vi "Parametros de adquisición texto para main.vi"(11 "Datos de Nueva Adquisición in":T1={"Montura"=enum."Motor Bipolar", "Equipo a Utilizar"=enum."TDS 2012B Osciloscope", "Datos Zaber"={"Sentido de Adquisición"=FALSE, "Comenzar Desde Home?"=FALSE, "Distancia a recorrer (cm)"=0, "Pasos motor"=0, "Distancia entre Lecturas (um)"=0.0, "Puerto"=""}, "Datos Bipolar/Unipolar"={"Puerto COM"="", "Pasos entre Lecturas"=0, "Numero de lecturas"=0, "Sentido del motor"=TRUE}, "Datos Archivo"={"Ruta Archivo"=path "", "Nombre de Prueba"=""}, "Datos actuales"={"Montura"="", "Equipo"="", "Posición Actual"="", "Distancia Total a recorrer"="", "distancia Entre lecturas"="", "Pasos entre lecturas"=""}, "Datos a Guardar In"={"Datos Cursor Tektronix"="", "Datos Lokin"="", "Posición Cero"=0.0, "Posición Actual"=0.0}, "Datos Osciloscopio"={"Sesión Visa Osciloscopio"="Tektronix_TDS2012C", "Tipo de Adquisición"=enum."Voltaje Pico Pico", "Canal a Utilizar"=enum."Canal 1", "Parametros de Adquisición"=enum."Una Muestra", "Número Promedio"=2}, "Datos Lock In"={"Visa Lock in"="Tektronix_TDS2012C"}} {"Datos Osciloscopio"."Número Promedio" min=2 max=20; "Datos a Guardar In"."Posición Actual" format="%#_10f"; "Datos a Guardar In"."Posición Cero" format="%#_10f"; "Datos Bipolar/Unipolar"."Numero de lecturas" max=910098 step=1}) -> (2 "Datos de Nueva Adquisición out":T1={"Montura"=enum."Motor Bipolar", "Equipo a Utilizar"=enum."TDS 2012B Osciloscope", "Datos Zaber"={"Sentido de Adquisición"=FALSE, "Comenzar Desde Home?"=FALSE, "Distancia a recorrer (cm)"=0, "Pasos motor"=0, "Distancia entre Lecturas (um)"=0.0, "Puerto"=""}, "Datos Bipolar/Unipolar"={"Puerto COM"="", "Pasos entre Lecturas"=0, "Numero de lecturas"=0, "Sentido del motor"=TRUE}, "Datos Archivo"={"Ruta Archivo"=path "", "Nombre de Prueba"=""}, "Datos actuales"={"Montura"="", "Equipo"="", "Posición Actual"="", "Distancia Total a recorrer"="", "distancia Entre lecturas"="", "Pasos entre lecturas"=""}, "Datos a Guardar In"={"Datos Cursor Tektronix"="", "Datos Lokin"="", "Posición Cero"=0.0, "Posición Actual"=0.0}, "Datos Osciloscopio"={"Sesión Visa Osciloscopio"="Tektronix_TDS2012C", "Tipo de Adquisición"=enum."Voltaje Pico Pico", "Canal a Utilizar"=enum."Canal 1", "Parametros de Adquisición"=enum."Una Muestra", "Número Promedio"=2}, "Datos Lock In"={"Visa Lock in"="Tektronix_TDS2012C"}} {"Datos Osciloscopio"."Número Promedio" min=2 max=20; "Datos a Guardar In"."Posición Actual" format="%#_10f"; "Datos a Guardar In"."Posición Cero" format="%#_10f"; "Datos Bipolar/Unipolar"."Numero de lecturas" max=910098 step=1})   [LabVIEW 2017]
uses:
  Type Definitions/Asistente de adquisicion Cluster.ctl
  Type Definitions/Datos Zaber.ctl
  Type Definitions/parametros motores.ctl
  Type Definitions/Datos a Guardar.ctl
  Type Definitions/datos osciloscopio.ctl
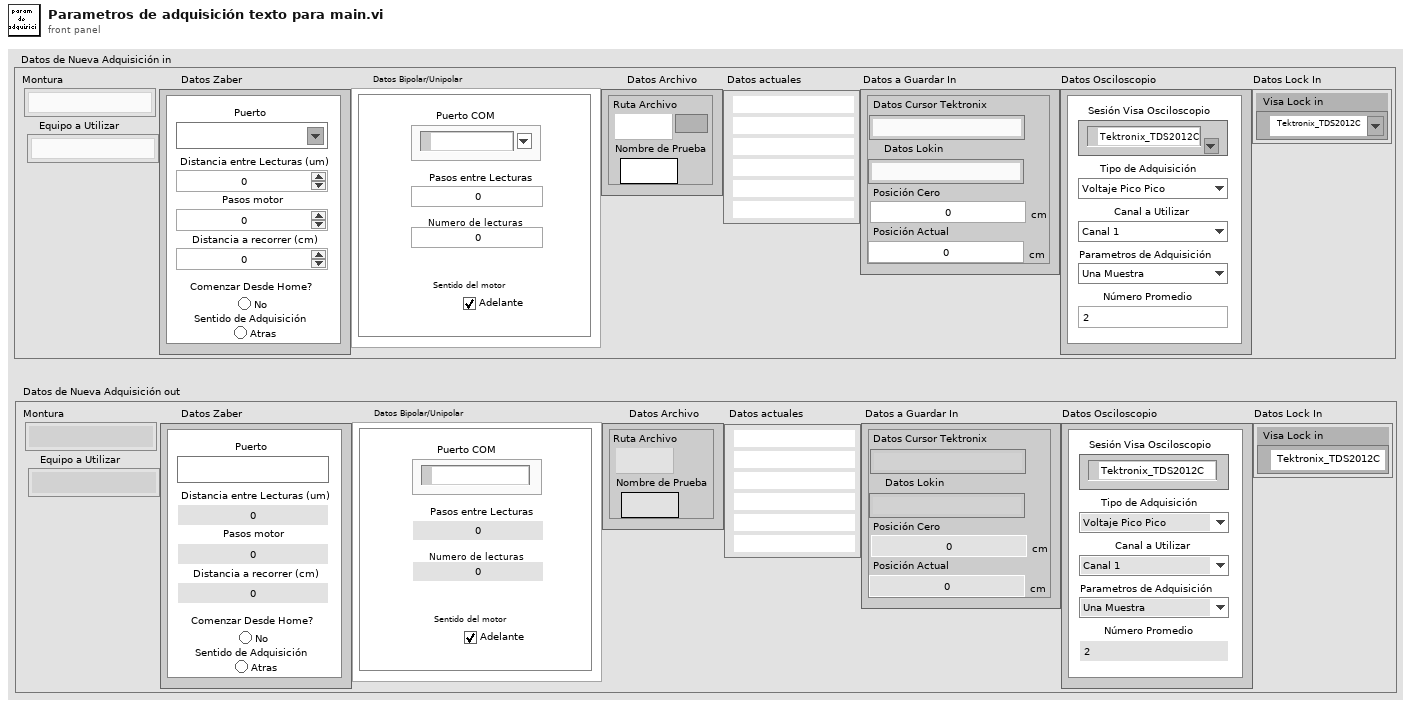
[diagram p1: front panel]
types:
  T1 = typedef "Asistente de adquisicion Cluster.ctl" = cluster{"Montura":enum16{"Zaber T-LSR450B", "Motor Bipolar", "Motor Unipolar"}, "Equipo a Utilizar":enum16{"SR830 Lock In", "TDS 2012B Osciloscope"}, "Datos Zaber":T2, "Datos Bipolar/Unipolar":T3, "Datos Archivo":cluster{"Ruta Archivo":path, "Nombre de Prueba":string}, "Datos actuales":cluster{"Montura":string, "Equipo":string, "Posición Actual":string, "Distancia Total a recorrer":string, "distancia Entre lecturas":string, "Pasos entre lecturas":string}, "Datos a Guardar In":T4, "Datos Osciloscopio":T5, "Datos Lock In":cluster{"Visa Lock in":refnum<visa-resource-name>}}
  T2 = typedef "Datos Zaber.ctl" = cluster{"Sentido de Adquisición":bool, "Comenzar Desde Home?":bool, "Distancia a recorrer (cm)":u32, "Pasos motor":i32, "Distancia entre Lecturas (um)":dbl, "Puerto":refnum<visa-resource-name>}
  T3 = typedef "parametros motores.ctl" = cluster{"Puerto COM":refnum<visa-resource-name>, "Pasos entre Lecturas":u16, "Numero de lecturas":u32, "Sentido del motor":bool}
  T4 = typedef "Datos a Guardar.ctl" = cluster{"Datos Cursor Tektronix":string, "Datos Lokin":string, "Posición Cero":dbl[unit], "Posición Actual":dbl[unit]}
  T5 = typedef "datos osciloscopio.ctl" = cluster{"Sesión Visa Osciloscopio":refnum<visa-resource-name>, "Tipo de Adquisición":enum16{"Voltaje Pico Pico", "Voltaje RMS", "Cursor Tiempo"}, "Canal a Utilizar":enum16{"Canal 1", "Canal 2", "Canal 1 y 2"}, "Parametros de Adquisición":enum16{"Una Muestra", "Promedio"}, "Número Promedio":i32}
  T6 = cluster{"Montura":string, "Equipo":string, "Posición Actual":string, "Distancia Total a recorrer":string, "distancia Entre lecturas":string, "Pasos entre lecturas":string}
  T7 = enum16{"Zaber T-LSR450B", "Motor Bipolar", "Motor Unipolar"}
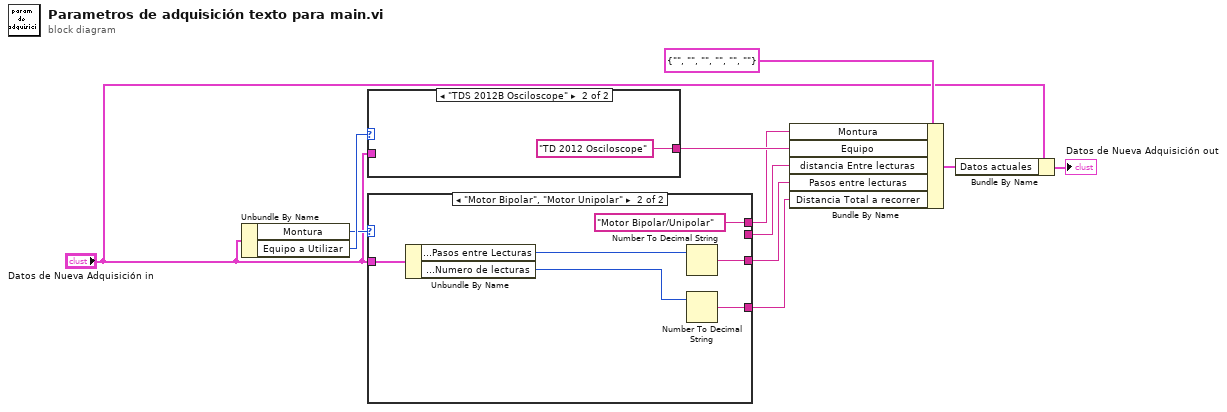
[diagram p0: block diagram]
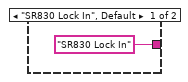
[diagram p2: hidden frame]
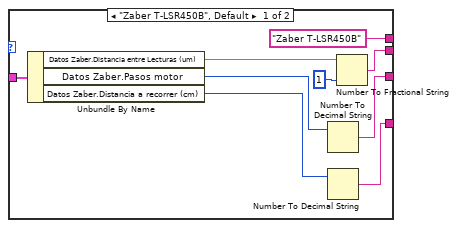
[diagram p3: hidden frame]
diagram:
  n1 = Unbundle By Name("Datos de Nueva Adquisición in") -> ("Montura"=w4:T7, "Equipo a Utilizar"=w5:enum16{"SR830 Lock In", "TDS 2012B Osciloscope"})
  n2 = case shown="\"TDS 2012B Osciloscope\"" w5 {
    tunnel: "Datos de Nueva Adquisición in" -> [_ _]
    tunnel: ["SR830 Lock In" "TD 2012 Osciloscope"] -> w8
    frame "SR830 Lock In", Default {
    }
    frame "TDS 2012B Osciloscope" {
    }
  }
  n3 = case shown="\"Motor Bipolar\", \"Motor Unipolar\"" w4 {
    tunnel: "Datos de Nueva Adquisición in" -> [w21 w27]
    tunnel: ["Zaber T-LSR450B" "Motor Bipolar/Unipolar"] -> w7
    tunnel: [w19 _] -> w9
    tunnel: [w17 w25] -> w10
    tunnel: [w15 w23] -> w11
    frame "Zaber T-LSR450B", Default {
      n4 = Unbundle By Name(w21) -> ("Datos Zaber.Distancia entre Lecturas (um)"=w20:dbl, "Datos Zaber.Pasos motor"=w18:i32, "Datos Zaber.Distancia a recorrer (cm)"=w16:u32)
      n5 = Number To Decimal String(number=w18) -> (decimal integer string=w17:string)  [unwired: 1 in]
      n6 = Number To Decimal String(number=w16) -> (decimal integer string=w15:string)  [unwired: 1 in]
      n7 = Number To Fractional String(number=w20, precision (6)=i16 1) -> (F-format string=w19:string)  [unwired: 2 in]
    }
    frame "Motor Bipolar", "Motor Unipolar" {
      n8 = Unbundle By Name(w27) -> ("Datos Bipolar/Unipolar.Pasos entre Lecturas"=w26:u16, "Datos Bipolar/Unipolar.Numero de lecturas"=w24:u32)
      n9 = Number To Decimal String(number=w26) -> (decimal integer string=w25:string)  [unwired: 1 in]
      n10 = Number To Decimal String(number=w24) -> (decimal integer string=w23:string)  [unwired: 1 in]
    }
  }
  n11 = Bundle By Name(cluster=T6 {"Montura"="", "Equipo"="", "Posición Actual"="", "Distancia Total a recorrer"="", "distancia Entre lecturas"="", "Pasos entre lecturas"=""} ("Datos actuales"), "Montura"=w7, "Equipo"=w8, "distancia Entre lecturas"=w9, "Pasos entre lecturas"=w10, "Distancia Total a recorrer"=w11) -> (w1:T6)
  n12 = Bundle By Name(cluster="Datos de Nueva Adquisición in", "Datos actuales"=w1) -> (→"Datos de Nueva Adquisición out":T1)
